vi "DeviationFinder.vi"(8 "Z":dbl, 9 "Y":dbl, 10 "X":dbl, 11 "Array in":dbl[][](array[numeric])) -> (0 "SD Z":dbl, 1 "SD Y":dbl, 2 "SD X":dbl, 3 "Array out":dbl[][](array[numeric]))   [LabVIEW 2020]
uses:
  <vilib>/Analysis/NI_AALBase.lvlib
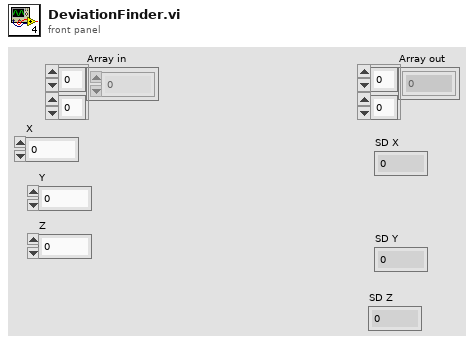
[diagram p1: front panel]
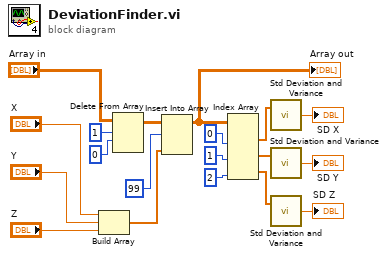
[diagram p0: block diagram]
diagram:
  n1 = Build Array("X", "Y", "Z") -> (w4:dbl[])
  n2 = Delete From Array(array="Array in", length=1, index (row)=0) -> (array with subset deleted=w17:dbl[][])  [unwired: 1 in, 1 out]
  n3 = Insert Into Array(array=w17, index (row)=99, new element=w4) -> (w19:dbl[][])  [unwired: 1 in]
  "Array out" <- w19
  n4 = Index Array(array=w19, index (col) #1=0 ("index"), index (col) #2=1 ("index"), index (col) #3=2 ("index (col)")) -> (element #1=w8:dbl[], element #2=w9:dbl[], element #3=w10:dbl[])  [unwired: 3 in]
  n5 = call <vilib>:"Std Deviation and Variance.vi"("X"=w8) -> ("standard deviation"=→"SD X":dbl)  [unwired: 1 in, 2 out]
  n6 = call <vilib>:"Std Deviation and Variance.vi"("X"=w9) -> ("standard deviation"=→"SD Y":dbl)  [unwired: 1 in, 2 out]
  n7 = call <vilib>:"Std Deviation and Variance.vi"("X"=w10) -> ("standard deviation"=→"SD Z":dbl)  [unwired: 1 in, 2 out]
